vi "Score_For_Active_Calls.vi"(8 "error in (no error)":errorcluster, 11 "Car Calls for Each Floor":T1) -> (0 "error out":errorcluster, 3 "Score":i32)   [LabVIEW 2026]
uses:
  Controls/Car_Calls_Status.ctl
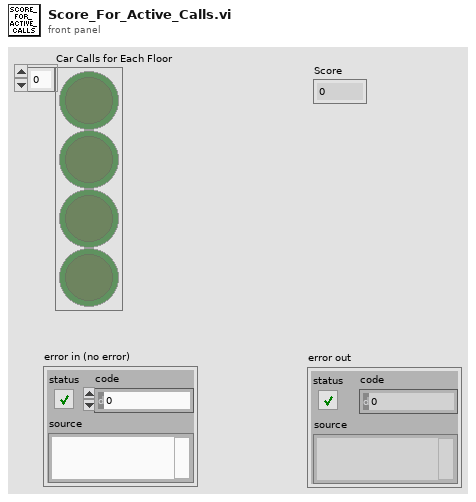
[diagram p1: front panel]
types:
  T1 = typedef "Car_Calls_Status.ctl" = bool[]
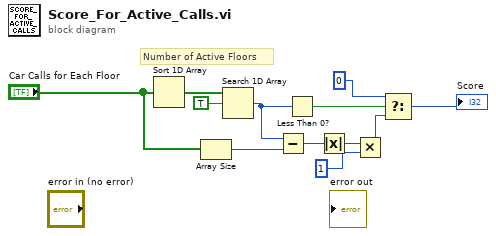
[diagram p0: block diagram]
diagram:
  # "Number of Active Floors"
  n1 = Sort 1D Array(array="Car Calls for Each Floor") -> (sorted array=w4:T1)
  n2 = Array Size(array="Car Calls for Each Floor") -> (size(s)=w2:i32)
  n3 = Search 1D Array(1D array=w4, element=TRUE) -> (index of element=w7:i32)  [unwired: 1 in]
  n4 = Subtract(x=w7, y=w2) -> (x-y=w8:i32)
  n5 = Less Than 0?(x=w7) -> (x < 0?=w6:bool)
  n6 = Absolute Value(x=w8) -> (abs(x)=w9:i32)
  n7 = Multiply(x=w9, y=1) -> (x*y=w10:i32)
  n8 = Select(t=0 ("y"), s=w6, f=w10) -> (s? t:f=→"Score":i32)
